vi "Untitled 2.vi"() -> ()   [LabVIEW 2012]
uses:
  Global1.vi
  <vilib>/Utility/file.llb/Read From Spreadsheet File (string).vi
panel:
  out "appended array":string[](array[string])
  out "error out":errorcluster
  out "Output":string
  out "OK":bool
  out "element":string
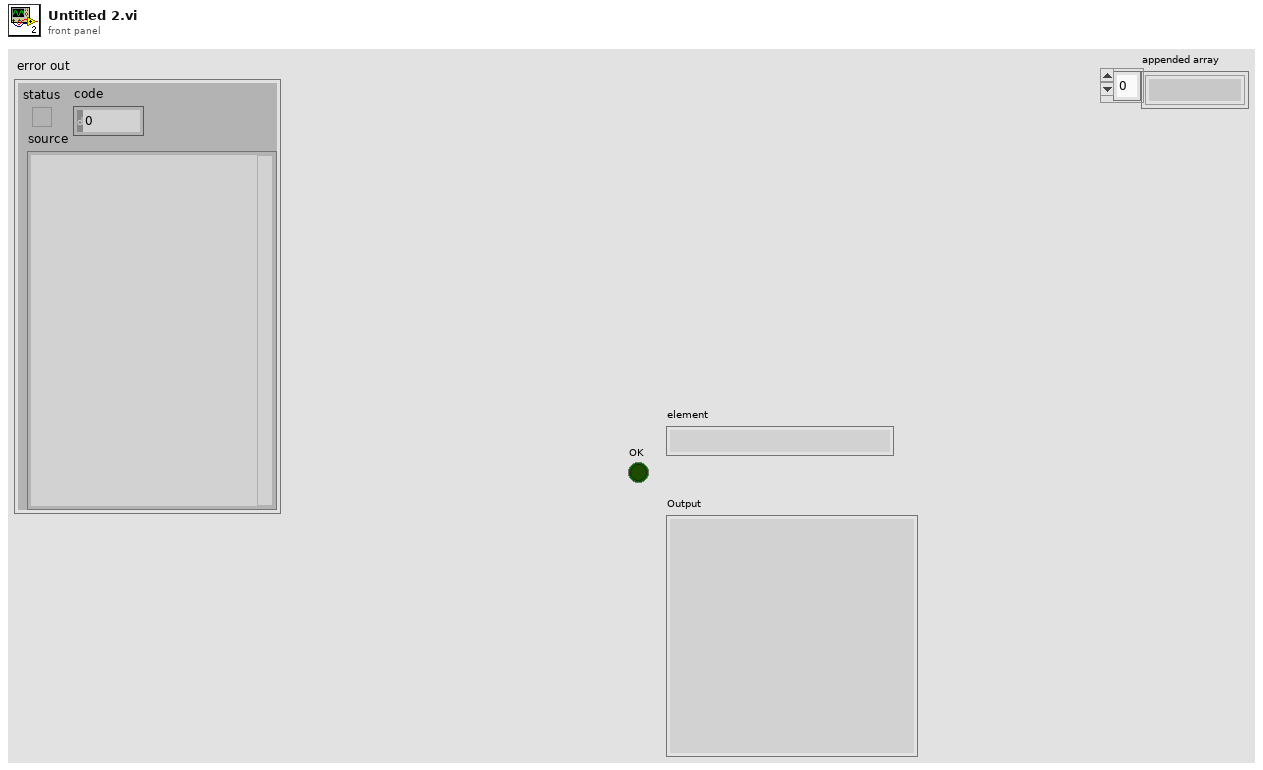
[diagram p1: front panel]
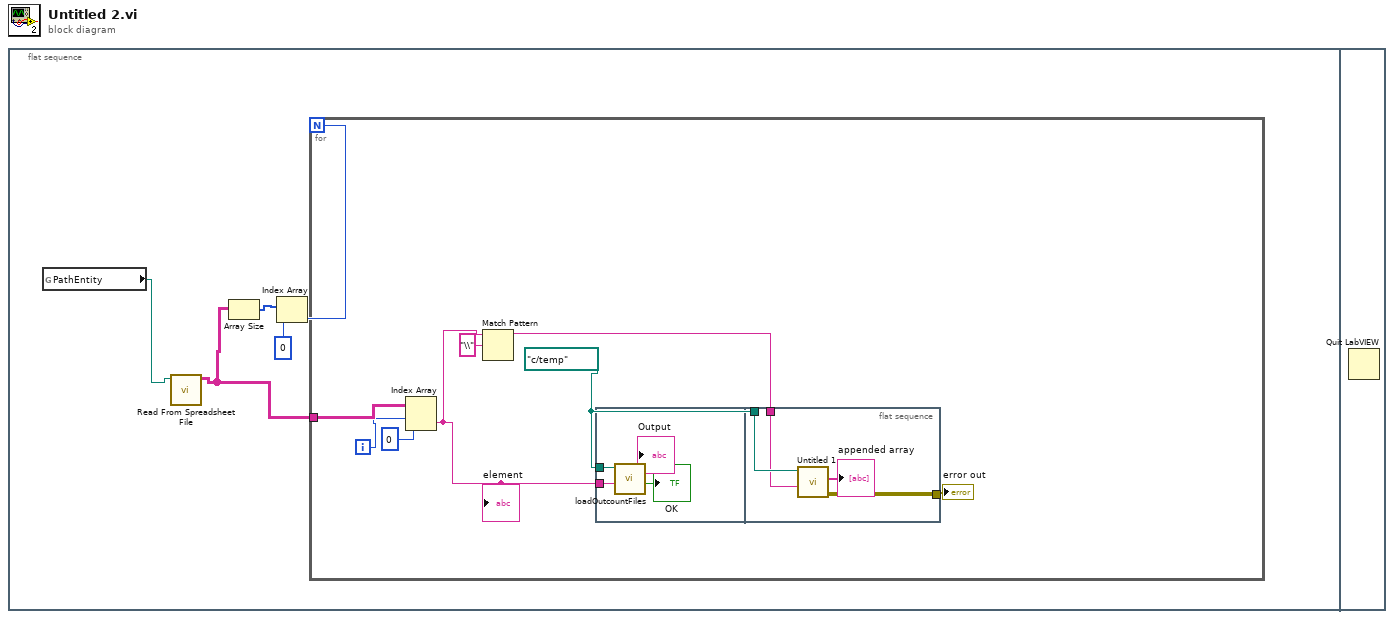
[diagram p0: block diagram]
diagram:
  n1 = flat-sequence {
    frame #0 {
      n2 = global read "Global1.vi" "PathEntity"() -> (w1:path)
      n3 = call-poly <vilib>:"Read From Spreadsheet File.vi"("file path (dialog if empty)"=w1) -> ("all rows"=w2:string[][])  [unwired: 6 in, 4 out]
      n4 = Array Size(array=w2) -> (size(s)=w5:i32[])
      n5 = Index Array(array=w5, index=0) -> (element=w3:i32)
      n6 = for {
        N: w3 -> [_]
        tunnel: w2 -> [w13]
        i -> [w11]
        w8 = path "c:/temp" ("working directory")
        n7 = Index Array(array=w13, index (row)=w11, index (col)=0 ("disabled index (col)")) -> (element=w9:string)
        "element" <- w9
        n8 = Match Pattern(string=w9, regular expression="\\") -> (before substring=w7:string)  [unwired: 1 in, 3 out]
        n9 = flat-sequence {
          tunnel: w9 -> [w17]
          tunnel: w8 -> [w16]
          tunnel: w8 -> [w21]
          tunnel: w7 -> [w20]
          tunnel: [w19] -> w6
          frame #0 {
            n10 = call "loadOutcountFiles.vi"("folder"=w17, "working directory"=w16) -> ("OK"=→"OK":bool, "Output"=→"Output":string)  [unwired: 8 in]
          }
          frame #1 {
            n11 = call "Untitled 1.vi"("machine"=w20, "base path"=w21) -> ("error out"=w19:errorcluster, "appended array"=→"appended array":string[])  [unwired: 8 in]
          }
        }
        "error out" <- w6
      }
    }
    frame #1 {
      n12 = Quit LabVIEW() -> ()  [unwired: 1 in]
    }
  }
